vi "GFGmultipleGet.vi"(7 "GFG Refnum (use when calling from external project)":refnum<vi>, 8 "error in (no error)":errorcluster, 11 "comma separated\nvariable names":string) -> (0 "error out":errorcluster, 3 "Array of Clusters of Variables":T2(array[cluster]))   [LabVIEW 2017, in "GFG library.lvlib"]
doc: "SciScan 1.2 160622"
uses:
  GFG library.lvlib
  <vilib>/Utility/VariantDataType/Type.ctl
  <vilib>/Utility/VariantDataType/VariantType.lvlib
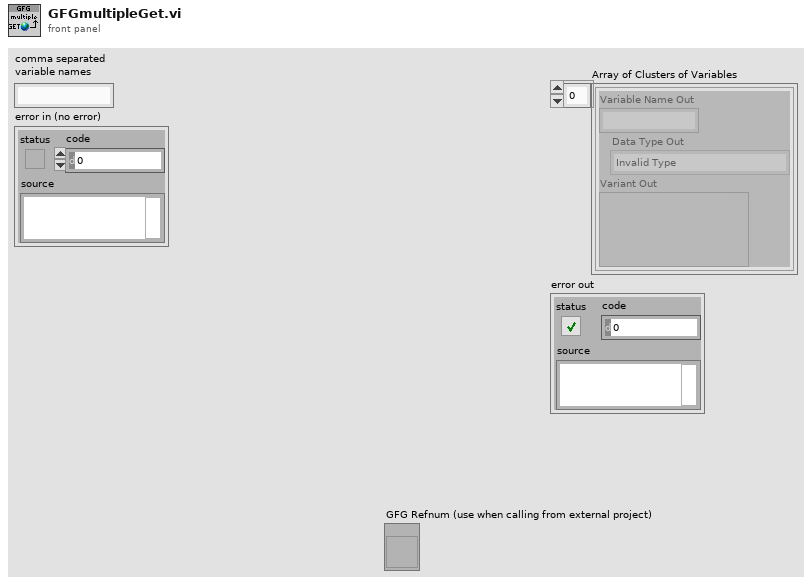
[diagram p1: front panel]
types:
  T1 = typedef "VariantType.lvlib/Type.ctl" = enum8{"Invalid Type", "Void", "I8", "I16", "I32", "I64", "U8", "U16", "U32", "U64", "Single Float", "Double Float", "Extended Float", "Single Complex", "Double Complex", "Extended Complex", "Enum U8", "Enum U16", "Enum U32", "Enum U64", "Single Float With Unit", "Double Float With Unit", "Extended Float With Unit", "Single Complex with Unit", "Double Complex with Unit", "Extended Complex with Unit", "Boolean", "String", "Path", "Picture", "Tag", "Array", "Cluster", "Variant", "LV Variant", "Waveform", "Timestamp", "Digital Waveform", "Digital Data", "ExpressData", "Refnum", "External Data", "VI", "Poly VI", "LabVIEW Class Instance", "Fixed Point"}
  T2 = cluster{"Variable Name Out":string, "Data Type Out":T1, "Variant Out":variant}[]
  T3 = cluster{"Variable Name Out":string, "Data Type Out":T1, "Variant Out":variant}
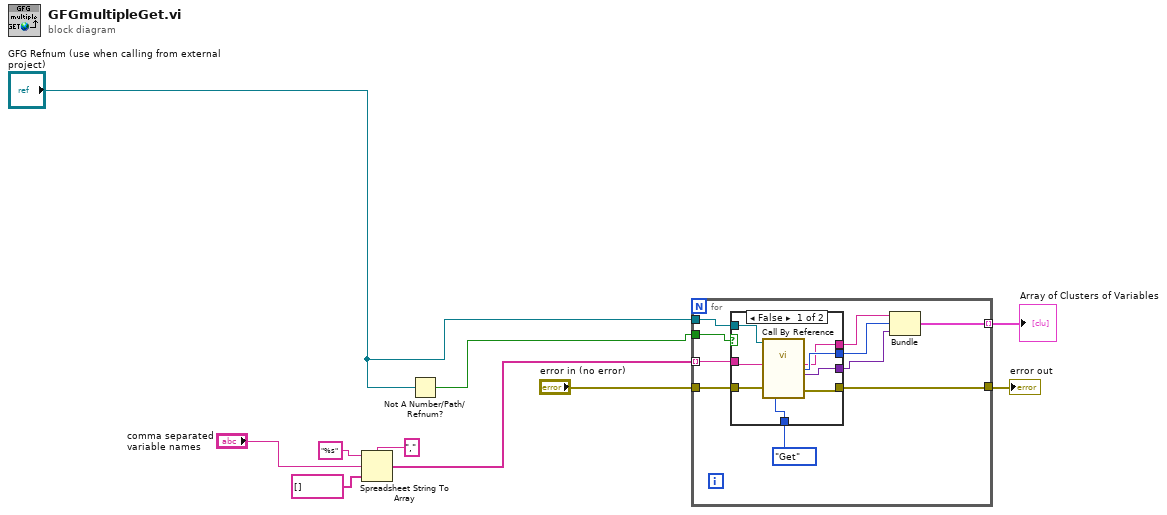
[diagram p0: block diagram]
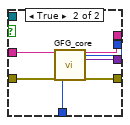
[diagram p2: hidden frame]
diagram:
  n1 = Spreadsheet String To Array(delimiter (Tab)=",", format string="%s" ("Variable Name in"), spreadsheet string="comma separated\nvariable names", array type (2D Dbl)=string[] [] ("Array")) -> (array=w5:string[])
  n2 = Not A Number/Path/Refnum?(number/path/refnum="GFG Refnum (use when calling from external project)") -> (NaN/Path/Refnum?=w6:bool)
  n3 = for {
    tunnel: w5 -> [w19] mode=indexing
    tunnel: "error in (no error)" -> [w18]
    tunnel: [w17] -> w3
    tunnel: [w13] -> w2 mode=indexing
    tunnel: w6 -> [w12]
    tunnel: "GFG Refnum (use when calling from external project)" -> [w11]
    n4 = case shown="False" w12 {
      tunnel: enum16{"Init", "Set", "Get"}."Get" ("Action") -> [w22 w35]
      tunnel: w19 -> [w23 w34]
      tunnel: w18 -> [w28 w33]
      tunnel: [w27 w32] -> w17
      tunnel: [w24 w31] -> w16
      tunnel: [w25 w30] -> w15
      tunnel: [w26 w29] -> w14
      tunnel: w11 -> [w21 _]
      frame False {
        n5 = call-by-ref "?"(reference=w21, "Variable Name in"=w23, "error in (no error)"=w28, "Action"=w22) -> ("Variable Name Out"=w24:string, "Data Type Out"=w25:T1, "Variant Out"=w26:variant, "error out"=w27:errorcluster)  [unwired: 11 in, 5 out]
      }
      frame True {
        n6 = call "GFG_core.vi"("Variable Name in"=w34, "error in (no error)"=w33, "Action"=w35) -> ("Variable Name Out"=w31:string, "Data Type Out"=w30:T1, "Variant Out"=w29:variant, "error out"=w32:errorcluster)  [unwired: 10 in, 3 out]
      }
    }
    n7 = Bundle("Variable Name Out"=w16, "Data Type Out"=w15, "Variant Out"=w14) -> (w13:T3)  [unwired: 1 in]
  }
  "error out" <- w3
  "Array of Clusters of Variables" <- w2
